vi "ready to sample.vi"(4 "error in (no error)":errorcluster) -> (0 "error out":errorcluster)   [LabVIEW 2010]
panel:
  out "message":string
  in  "?":bool
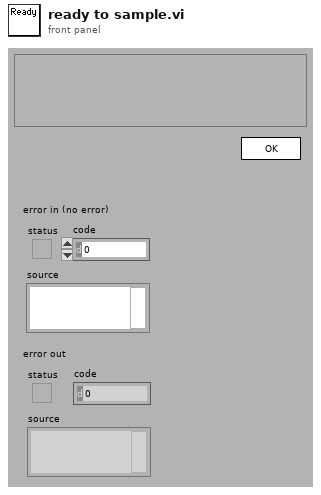
[diagram p1: front panel]
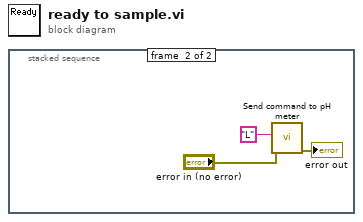
[diagram p0: block diagram]
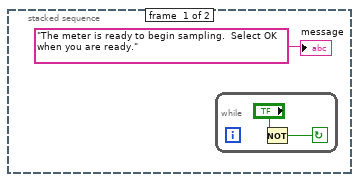
[diagram p2: hidden frame]
diagram:
  n1 = stacked-sequence {
    frame #0 {
      n2 = while {
        stop <- w2 continue-if-true
        n3 = Not(x="?") -> (.not. x?=w2:bool)
      }
      "message" <- "The meter is ready to begin sampling.  Select OK when you are ready."
    }
    frame #1 {
      n4 = call "Send command to pH meter"("error in (no error)"="error in (no error)", "string to write"="L") -> ("error out"=→"error out":errorcluster)  [unwired: 8 in, 1 out]
    }
  }
